vi "Angle Between Vectors.vi"(1 "B":cluster{"x":dbl, "y":dbl}, 2 "A":cluster{"x":dbl, "y":dbl}) -> (0 "Angle (rads)":dbl)   [LabVIEW 2011]
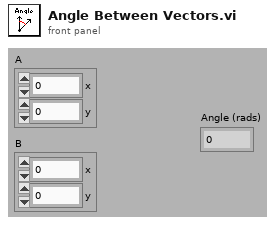
[diagram p1: front panel]
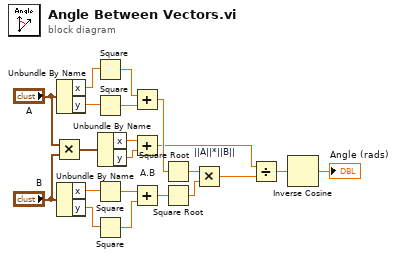
[diagram p0: block diagram]
diagram:
  n1 = Multiply(x="A", y="B") -> (x*y=w21:cluster{"x":dbl, "y":dbl})
  n2 = Unbundle By Name("A") -> ("x"=w18:dbl, "y"=w17:dbl)
  n3 = Unbundle By Name("B") -> ("x"=w16:dbl, "y"=w15:dbl)
  n4 = Square(x=w18) -> (x^2=w12:dbl)
  n5 = Square(x=w17) -> (x^2=w11:dbl)
  n6 = Square(x=w16) -> (x^2=w13:dbl)
  n7 = Square(x=w15) -> (x^2=w14:dbl)
  n8 = Unbundle By Name(w21) -> ("x"=w20:dbl, "y"=w19:dbl)
  n9 = Add(x=w12, y=w11) -> (x+y=w10:dbl)
  n10 = Add "A.B"(x=w20, y=w19) -> (x+y=w6:dbl)
  n11 = Add(x=w13, y=w14) -> (x+y=w9:dbl)
  n12 = Square Root(x=w10) -> (sqrt(x)=w8:dbl)
  n13 = Square Root(x=w9) -> (sqrt(x)=w7:dbl)
  n14 = Multiply "||A||*||B||"(x=w8, y=w7) -> (x*y=w5:dbl)
  n15 = Divide(x=w6, y=w5) -> (x/y=w4:dbl)
  n16 = Inverse Cosine(1:w4) -> (0:→"Angle (rads)":dbl)
